vi "Untitled 1.vi"() -> ()   [LabVIEW 2024]
panel:
  in  ".NET Container":refnum<k24>(container)
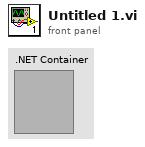
[diagram p1: front panel]
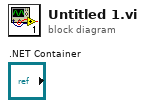
[diagram p0: block diagram]
diagram:
